vi "Log Config.vi"(0 "Log File Ref In":refnum<file>, 2 "Measurement Config Ref.":refnum<vi>, 11 "error in":errorcluster) -> (4 "Log File Ref Out":refnum<file>, 6 "Cancelled":bool, 15 "error out":errorcluster)   [LabVIEW 2024, in "dataLogger.lvlib"]
doc: "<B>Log Measurment Configuration</B> API. \n\nGets Measurment config. cluster and log the setting in CSV format."
uses:
  dataLogger.lvlib
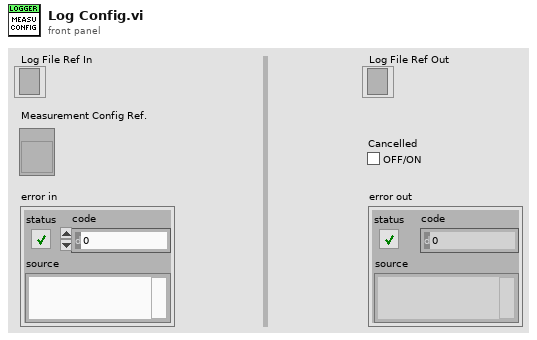
[diagram p1: front panel]
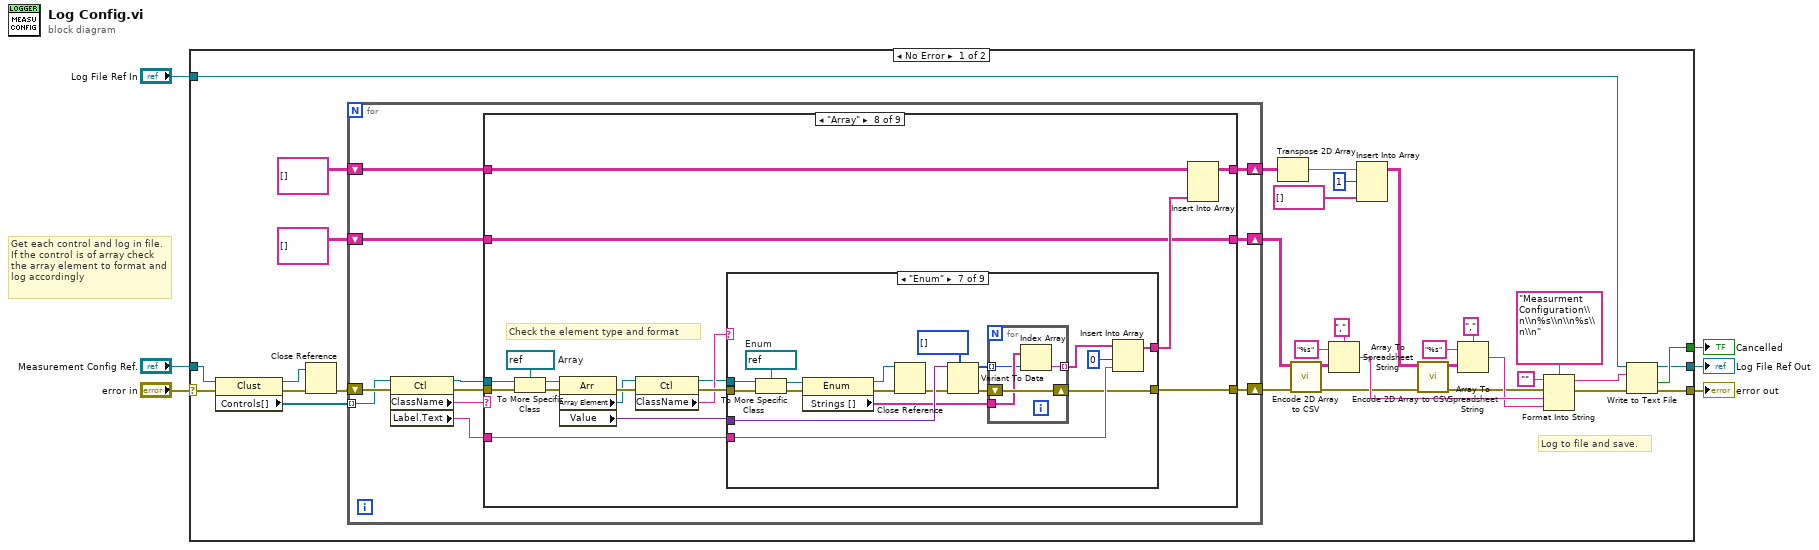
[diagram p0: block diagram]
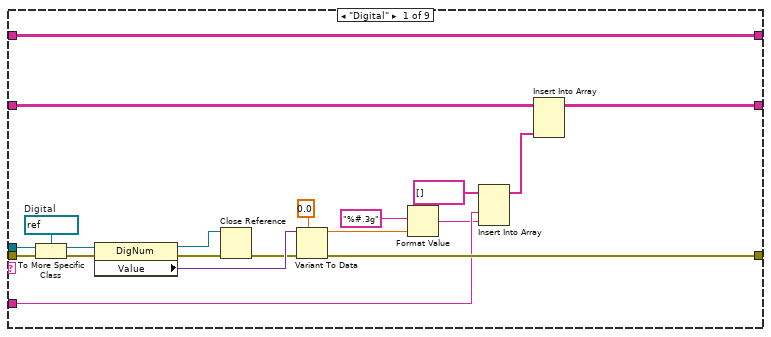
[diagram p2: hidden frame]
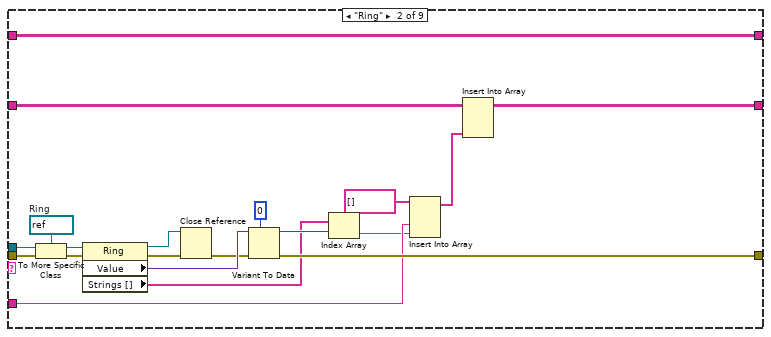
[diagram p3: hidden frame]
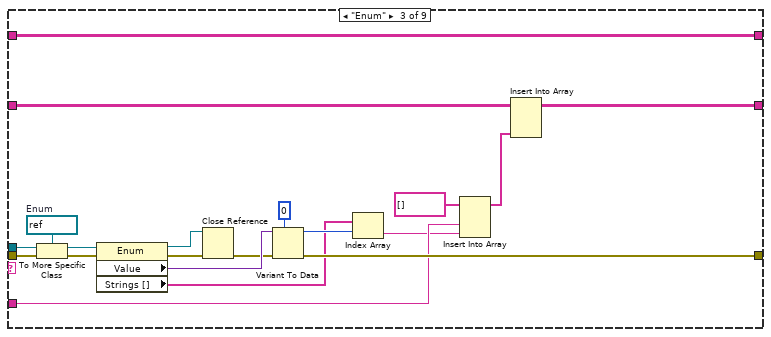
[diagram p4: hidden frame]
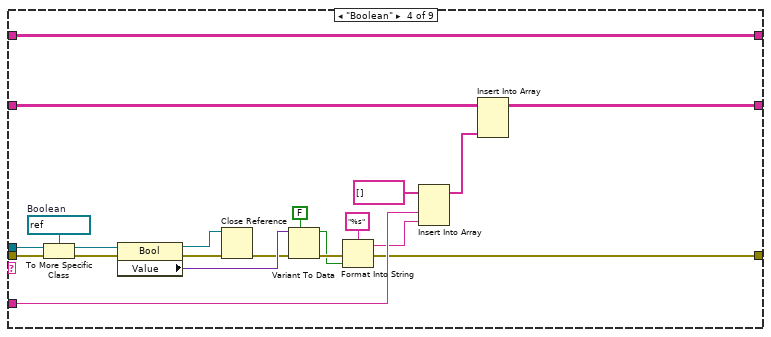
[diagram p5: hidden frame]
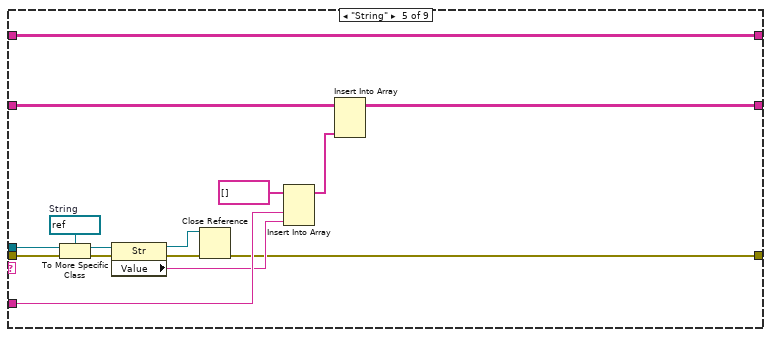
[diagram p6: hidden frame]
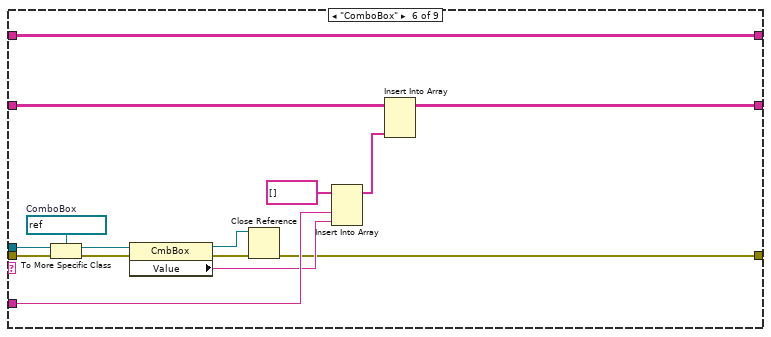
[diagram p7: hidden frame]
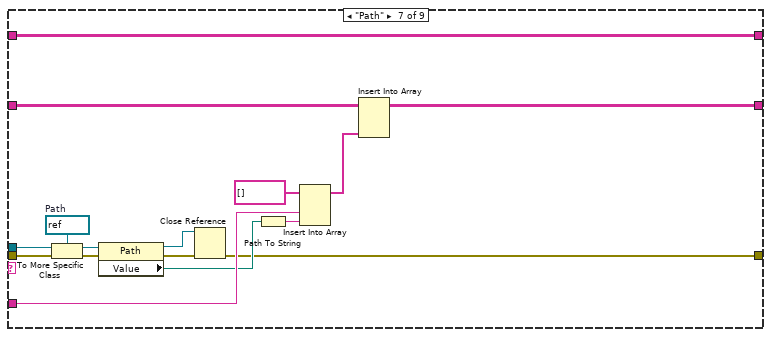
[diagram p8: hidden frame]
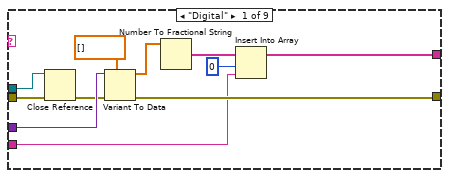
[diagram p9: hidden frame]
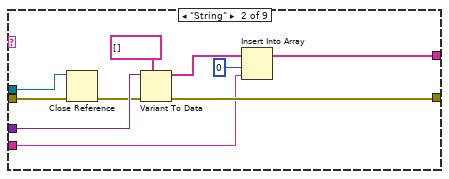
[diagram p10: hidden frame]
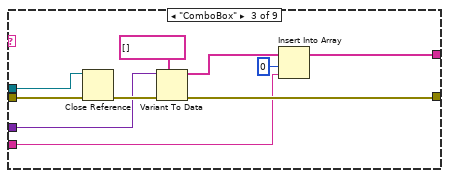
[diagram p11: hidden frame]
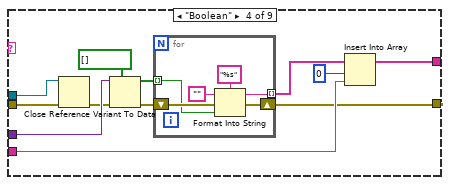
[diagram p12: hidden frame]
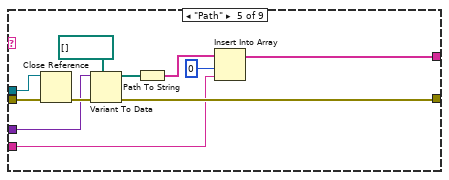
[diagram p13: hidden frame]
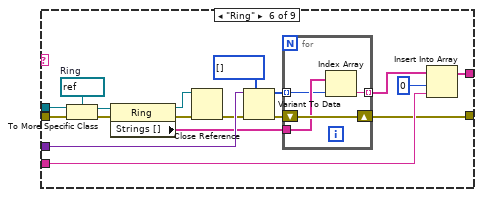
[diagram p14: hidden frame]
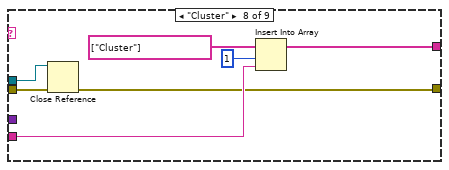
[diagram p15: hidden frame]
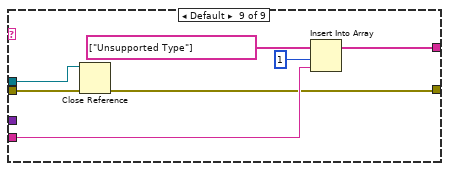
[diagram p16: hidden frame]
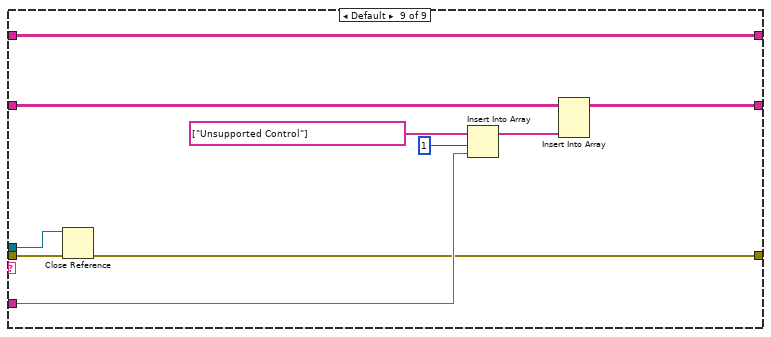
[diagram p17: hidden frame]
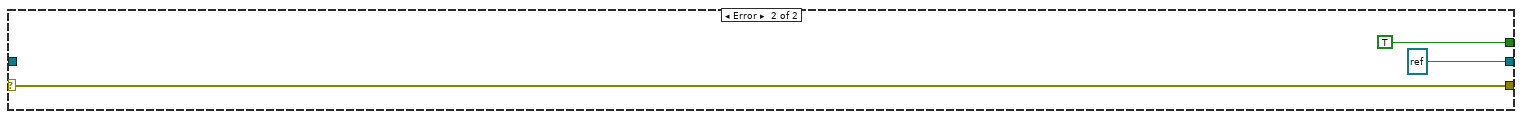
[diagram p18: hidden frame]
diagram:
  # "Get each control and log in file. If the control is of array check the array element to format and log accordingly"
  n1 = case shown="No Error" "error in" {
    selector: "error in" -> [w36 w325]
    tunnel: "Measurement Config Ref." -> [w39 _]
    tunnel: [w21 w325] -> w5
    tunnel: [w20 TRUE ("cancelled")] -> w3
    tunnel: "Log File Ref In" -> [w17 _]
    tunnel: [w16 refnum<file> refnum ("refnum out")] -> w1
    frame No Error {
      # "Log to file and save."
      n2 = property class="Clust"(reference=w39, error in=w36) -> (reference out=w23:refnum<vi>, error out=w37:errorcluster, "Controls[]"=w38:refnum<vi>[])
      n3 = Close Reference(reference=w23, error in (no error)=w37) -> (error out=w24:errorcluster)
      n4 = for {
        tunnel: w38 -> [w47] mode=indexing
        shift-right: [w49] -> w13
        shift-left: w24 -> [w50]
        shift-right: [w46] -> w34
        shift-left: string[][] [] ("Pin Config Data") -> [w45]
        shift-right: [w41] -> w10
        shift-left: string[][] [] ("General Setting") -> [w42]
        n5 = property class="Ctl"(reference=w47, error in=w50) -> (reference out=w40:refnum<vi>, error out=w48:errorcluster, "ClassName"=w44:string, "Label.Text"=w43:string)
        n6 = case shown="\"Array\"" w44 {
          tunnel: [w64 w84 w104 w117 w133 w150 w164 w193 w314] -> w49
          tunnel: w48 -> [w70 w90 w110 w131 w146 w161 w177 w194 w322]
          tunnel: [w69 w89 w109 w130 w145 w160 w176 w183 w321] -> w46
          tunnel: w45 -> [w69 w89 w109 w130 w145 w160 w176 w184 w321]
          tunnel: w43 -> [w58 w80 w100 w122 w139 w154 w171 w181 w316]
          tunnel: w42 -> [w56 w79 w99 w121 w138 w153 w170 w179 w320]
          tunnel: [w55 w78 w98 w120 w137 w152 w169 w179 w319] -> w41
          tunnel: w40 -> [w53 w73 w93 w111 w134 w148 w162 w178 w313]
          frame "Digital" {
            w66 = refnum<vi> refnum  # Digital
            n7 = To More Specific Class(target class=w66, reference=w53, error in=w70) -> (specific class reference=w65:refnum<vi>, error out=w67:errorcluster)
            n8 = property class="DigNum"(reference=w65, error in=w67) -> (reference out=w51:refnum<vi>, error out=w68:errorcluster, "Value"=w62:variant)
            n9 = Close Reference(reference=w51, error in (no error)=w68) -> (error out=w52:errorcluster)
            n10 = Variant To Data(error in=w52, type=0.0, Variant=w62) -> (data=w60:dbl, error out=w64:errorcluster)
            n11 = Format Value(format string="%#.3g", value (0)=w60) -> (output string=w57:string)  [unwired: 1 in]
            n12 = Insert Into Array(array=string[] [] ("General Settings"), new element #1=w58, new element #2=w57) -> (w54:string[])  [unwired: 1 in]
            n13 = Insert Into Array(array=w56, new element=w54) -> (w55:string[][])  [unwired: 2 in]
          }
          frame "Ring" {
            w86 = refnum<vi> refnum  # Ring
            n14 = To More Specific Class(target class=w86, reference=w73, error in=w90) -> (specific class reference=w85:refnum<vi>, error out=w87:errorcluster)
            n15 = property class="Ring"(reference=w85, error in=w87) -> (reference out=w71:refnum<vi>, error out=w88:errorcluster, "Value"=w82:variant, "Strings []"=w75:string[])
            n16 = Close Reference(reference=w71, error in (no error)=w88) -> (error out=w72:errorcluster)
            n17 = Variant To Data(error in=w72, type=0, Variant=w82) -> (data=w76:i32, error out=w84:errorcluster)
            n18 = Index Array(array=w75, index=w76) -> (element=w74:string)
            n19 = Insert Into Array(array=string[] [] ("General Settings"), new element #1=w80, new element #2=w74) -> (w77:string[])  [unwired: 1 in]
            n20 = Insert Into Array(array=w79, new element=w77) -> (w78:string[][])  [unwired: 2 in]
          }
          frame "Enum" {
            w106 = refnum<vi> refnum  # Enum
            n21 = To More Specific Class(target class=w106, reference=w93, error in=w110) -> (specific class reference=w105:refnum<vi>, error out=w107:errorcluster)
            n22 = property class="Enum"(reference=w105, error in=w107) -> (reference out=w91:refnum<vi>, error out=w108:errorcluster, "Value"=w102:variant, "Strings []"=w95:string[])
            n23 = Close Reference(reference=w91, error in (no error)=w108) -> (error out=w92:errorcluster)
            n24 = Variant To Data(error in=w92, type=0, Variant=w102) -> (data=w96:i32, error out=w104:errorcluster)
            n25 = Index Array(array=w95, index=w96) -> (element=w94:string)
            n26 = Insert Into Array(array=string[] [] ("General Settings"), new element #1=w100, new element #2=w94) -> (w97:string[])  [unwired: 1 in]
            n27 = Insert Into Array(array=w99, new element=w97) -> (w98:string[][])  [unwired: 2 in]
          }
          frame "Boolean" {
            w127 = refnum<vi> refnum  # Boolean
            n28 = To More Specific Class(target class=w127, reference=w111, error in=w131) -> (specific class reference=w126:refnum<vi>, error out=w128:errorcluster)
            n29 = property class="Bool"(reference=w126, error in=w128) -> (reference out=w112:refnum<vi>, error out=w129:errorcluster, "Value"=w124:variant)
            n30 = Close Reference(reference=w112, error in (no error)=w129) -> (error out=w113:errorcluster)
            n31 = Variant To Data(error in=w113, type=FALSE, Variant=w124) -> (data=w116:bool, error out=w125:errorcluster)
            n32 = Format Into String(format string="%s", error in=w125, w116) -> (resulting string=w114:string, error out=w117:errorcluster)  [unwired: 1 in]
            n33 = Insert Into Array(array=string[] [] ("General Settings"), new element #1=w122, new element #2=w114) -> (w119:string[])  [unwired: 1 in]
            n34 = Insert Into Array(array=w121, new element=w119) -> (w120:string[][])  [unwired: 2 in]
          }
          frame "String" {
            w142 = refnum<vi> refnum  # String
            n35 = To More Specific Class(target class=w142, reference=w134, error in=w146) -> (specific class reference=w141:refnum<vi>, error out=w143:errorcluster)
            n36 = property class="Str"(reference=w141, error in=w143) -> (reference out=w132:refnum<vi>, error out=w144:errorcluster, "Value"=w135:string)
            n37 = Close Reference(reference=w132, error in (no error)=w144) -> (error out=w133:errorcluster)
            n38 = Insert Into Array(array=string[] [] ("General Settings"), new element #1=w139, new element #2=w135) -> (w136:string[])  [unwired: 1 in]
            n39 = Insert Into Array(array=w138, new element=w136) -> (w137:string[][])  [unwired: 2 in]
          }
          frame "ComboBox" {
            w157 = refnum<vi> refnum  # ComboBox
            n40 = To More Specific Class(target class=w157, reference=w148, error in=w161) -> (specific class reference=w156:refnum<vi>, error out=w158:errorcluster)
            n41 = property class="CmbBox"(reference=w156, error in=w158) -> (reference out=w149:refnum<vi>, error out=w159:errorcluster, "Value"=w151:string)
            n42 = Close Reference(reference=w149, error in (no error)=w159) -> (error out=w150:errorcluster)
            n43 = Insert Into Array(array=string[] [] ("General Settings"), new element #1=w154, new element #2=w151) -> (w147:string[])  [unwired: 1 in]
            n44 = Insert Into Array(array=w153, new element=w147) -> (w152:string[][])  [unwired: 2 in]
          }
          frame "Path" {
            w174 = refnum<vi> refnum  # Path
            n45 = To More Specific Class(target class=w174, reference=w162, error in=w177) -> (specific class reference=w173:refnum<vi>, error out=w175:errorcluster)
            n46 = property class="Path"(reference=w173, error in=w175) -> (reference out=w163:refnum<vi>, error out=w165:errorcluster, "Value"=w167:path)
            n47 = Close Reference(reference=w163, error in (no error)=w165) -> (error out=w164:errorcluster)
            n48 = Path To String(path=w167) -> (string=w166:string)
            n49 = Insert Into Array(array=string[] [] ("General Settings"), new element #1=w171, new element #2=w166) -> (w168:string[])  [unwired: 1 in]
            n50 = Insert Into Array(array=w170, new element=w168) -> (w169:string[][])  [unwired: 2 in]
          }
          frame "Array" {
            w190 = refnum<vi> refnum  # Array
            # "Check the element type and format"
            n51 = To More Specific Class(target class=w190, reference=w178, error in=w194) -> (specific class reference=w191:refnum<vi>, error out=w192:errorcluster)
            n52 = property class="Arr"(reference=w191, error in=w192) -> (error out=w189:errorcluster, "Array Element"=w187:refnum<vi>, "Value"=w185:variant)  [unwired: 1 out]
            n53 = property class="Ctl"(reference=w187, error in=w189) -> (reference out=w180:refnum<vi>, error out=w188:errorcluster, "ClassName"=w186:string)
            n54 = case shown="\"Enum\"" w186 {
              tunnel: [w202 w212 w223 w232 w251 w261 w286 w300 w307] -> w193
              tunnel: w188 -> [w204 w213 w224 w236 w254 w272 w294 w302 w312]
              tunnel: w185 -> [w203 w214 w216 w235 w244 w271 w293 _ _]
              tunnel: [w197 w210 w221 w228 w249 w270 w292 w305 w310] -> w182
              tunnel: w181 -> [w199 w209 w220 w233 w248 w269 w291 w303 w311]
              tunnel: w180 -> [w195 w206 w217 w226 w245 w265 w289 w299 w306]
              frame "Digital" {
                n55 = Close Reference(reference=w195, error in (no error)=w204) -> (error out=w196:errorcluster)
                n56 = Variant To Data(error in=w196, type=dbl[] [], Variant=w203) -> (data=w201:dbl[], error out=w202:errorcluster)
                n57 = Number To Fractional String(number=w201) -> (F-format string=w200:string[])  [unwired: 3 in]
                n58 = Insert Into Array(array=w200, index=0, new element=w199) -> (w197:string[])
              }
              frame "String" {
                n59 = Close Reference(reference=w206, error in (no error)=w213) -> (error out=w207:errorcluster)
                n60 = Variant To Data(error in=w207, type=string[] [], Variant=w214) -> (data=w211:string[], error out=w212:errorcluster)
                n61 = Insert Into Array(array=w211, index=0, new element=w209) -> (w210:string[])
              }
              frame "ComboBox" {
                n62 = Close Reference(reference=w217, error in (no error)=w224) -> (error out=w218:errorcluster)
                n63 = Variant To Data(error in=w218, type=string[] [], Variant=w216) -> (data=w222:string[], error out=w223:errorcluster)
                n64 = Insert Into Array(array=w222, index=0, new element=w220) -> (w221:string[])
              }
              frame "Boolean" {
                n65 = Close Reference(reference=w226, error in (no error)=w236) -> (error out=w227:errorcluster)
                n66 = Variant To Data(error in=w227, type=bool[] [], Variant=w235) -> (data=w230:bool[], error out=w231:errorcluster)
                n67 = for {
                  shift-right: [w241] -> w232
                  shift-left: w231 -> [w242]
                  tunnel: w230 -> [w240] mode=indexing
                  tunnel: [w238] -> w229 mode=indexing
                  n68 = Format Into String(format string="%s", initial string="", error in=w242, w240) -> (resulting string=w238:string, error out=w241:errorcluster)
                }
                n69 = Insert Into Array(array=w229, index=0, new element=w233) -> (w228:string[])
              }
              frame "Path" {
                n70 = Close Reference(reference=w245, error in (no error)=w254) -> (error out=w246:errorcluster)
                n71 = Variant To Data(error in=w246, type=path[] [], Variant=w244) -> (data=w252:path[], error out=w251:errorcluster)
                n72 = Path To String(path=w252) -> (string=w250:string[])
                n73 = Insert Into Array(array=w250, index=0, new element=w248) -> (w249:string[])
              }
              frame "Ring" {
                w263 = refnum<vi> refnum  # Ring
                n74 = To More Specific Class(target class=w263, reference=w265, error in=w272) -> (specific class reference=w264:refnum<vi>, error out=w266:errorcluster)
                n75 = property class="Ring"(reference=w264, error in=w266) -> (reference out=w255:refnum<vi>, error out=w267:errorcluster, "Strings []"=w262:string[])
                n76 = Close Reference(reference=w255, error in (no error)=w267) -> (error out=w256:errorcluster)
                n77 = Variant To Data(error in=w256, type=i32[] [], Variant=w271) -> (data=w259:i32[], error out=w260:errorcluster)
                n78 = for {
                  tunnel: w262 -> [w275]
                  shift-right: [w276] -> w261
                  shift-left: w260 -> [w276]
                  tunnel: w259 -> [w274] mode=indexing
                  tunnel: [w273] -> w258 mode=indexing
                  n79 = Index Array(array=w275, index=w274) -> (element=w273:string)
                }
                n80 = Insert Into Array(array=w258, index=0, new element=w269) -> (w270:string[])
              }
              frame "Enum" {
                w287 = refnum<vi> refnum  # Enum
                n81 = To More Specific Class(target class=w287, reference=w289, error in=w294) -> (specific class reference=w288:refnum<vi>, error out=w290:errorcluster)
                n82 = property class="Enum"(reference=w288, error in=w290) -> (reference out=w277:refnum<vi>, error out=w284:errorcluster, "Strings []"=w283:string[])
                n83 = Close Reference(reference=w277, error in (no error)=w284) -> (error out=w278:errorcluster)
                n84 = Variant To Data(error in=w278, type=i32[] [], Variant=w293) -> (data=w281:i32[], error out=w282:errorcluster)
                n85 = for {
                  tunnel: w283 -> [w297]
                  shift-right: [w298] -> w286
                  shift-left: w282 -> [w298]
                  tunnel: w281 -> [w295] mode=indexing
                  tunnel: [w296] -> w280 mode=indexing
                  n86 = Index Array(array=w297, index=w295) -> (element=w296:string)
                }
                n87 = Insert Into Array(array=w280, index=0, new element=w291) -> (w292:string[])
              }
              frame "Cluster" {
                n88 = Close Reference(reference=w299, error in (no error)=w302) -> (error out=w300:errorcluster)
                n89 = Insert Into Array(array=string[] ["Cluster"] ("Label.Text"), index=1, new element=w303) -> (w305:string[])
              }
              frame Default {
                n90 = Close Reference(reference=w306, error in (no error)=w312) -> (error out=w307:errorcluster)
                n91 = Insert Into Array(array=string[] ["Unsupported Type"] ("Label.Text"), index=1, new element=w311) -> (w310:string[])
              }
            }
            n92 = Insert Into Array(array=w184, new element=w182) -> (w183:string[][])  [unwired: 2 in]
          }
          frame Default {
            n93 = Close Reference(reference=w313, error in (no error)=w322) -> (error out=w314:errorcluster)
            n94 = Insert Into Array(array=string[] ["Unsupported Control"] ("new element/subarray"), index=1, new element=w316) -> (w317:string[])
            n95 = Insert Into Array(array=w320, new element=w317) -> (w319:string[][])  [unwired: 2 in]
          }
        }
      }
      n96 = Transpose 2D Array(2D array=w34) -> (transposed array=w32:string[][])
      n97 = call "Encode 2D Array to CSV.vi"("error in"=w13, "2D Array In"=w10) -> ("error out"=w12:errorcluster, "2D Array Out"=w9:string[][])  [unwired: 8 in]
      n98 = Array To Spreadsheet String(delimiter (Tab)=",", array=w9, 3:"%s" ("format string")) -> (spreadsheet string=w26:string)
      n99 = Insert Into Array(array=w32, index (row)=1, new element=string[] [] ("new element/subarray")) -> (w8:string[][])  [unwired: 1 in]
      n100 = call "Encode 2D Array to CSV.vi"("error in"=w12, "2D Array In"=w8) -> ("error out"=w11:errorcluster, "2D Array Out"=w7:string[][])  [unwired: 8 in]
      n101 = Array To Spreadsheet String(delimiter (Tab)=",", array=w7, 3:"%s" ("format string")) -> (spreadsheet string=w18:string)
      n102 = Format Into String(format string="Measurment Configuration\\n\\n%s\\n\\n%s\\n\\n", initial string="", error in=w11, w26, w18) -> (resulting string=w25:string, error out=w19:errorcluster)
      n103 = Write to Text File(file (use dialog)=w17, text=w25, error in=w19) -> (refnum out=w16:refnum<file>, cancelled=w20:bool, error out=w21:errorcluster)  [unwired: 1 in]
    }
    frame Error {
    }
  }
  "error out" <- w5
  "Cancelled" <- w3
  "Log File Ref Out" <- w1
